vi "Estimated Time Required.vi"(1 "Lithography Information":T1(array[cluster])) -> (0 "Estimated Time Required":timestamp format="%<%I:%M:%S>T")   [LabVIEW 2011]
doc: "Calculates the time required to complete lithography."
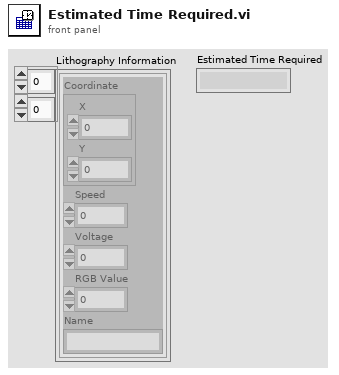
[diagram p1: front panel]
types:
  T1 = cluster{"Coordinate":cluster{"X":dbl, "Y":dbl}, "Speed":dbl, "Voltage":dbl, "RGB Value":i32, "Name":string}[][]
  T2 = cluster{"Coordinate":cluster{"X":dbl, "Y":dbl}, "Speed":dbl, "Voltage":dbl, "RGB Value":i32, "Name":string}
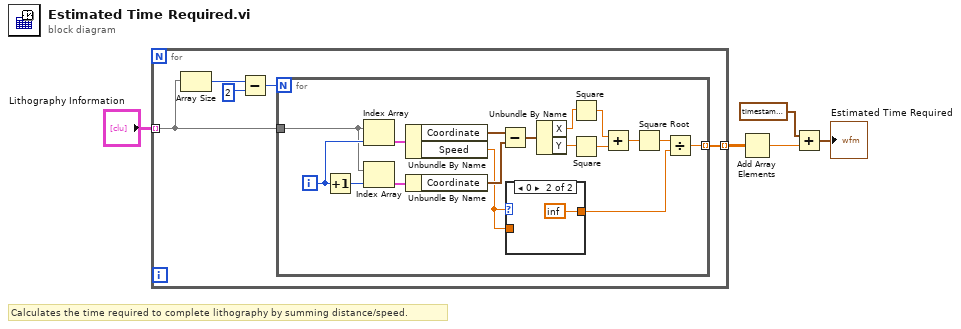
[diagram p0: block diagram]
diagram:
  # "Calculates the time required to complete lithography by summing distance/speed."
  n1 = for {
    tunnel: "Lithography Information" -> [w10] mode=indexing
    tunnel: [w9] -> w4 mode=indexing
    n2 = Array Size(array=w10) -> (size(s)=w7:i32)
    n3 = Subtract(x=w7, y=2) -> (x-y=w6:i32)
    n4 = for {
      N: w6 -> [_]
      tunnel: w10 -> [w25]
      tunnel: [w13] -> w9 mode=indexing
      i -> [w26]
      n5 = Increment(x=w26) -> (x+1=w27:i32)
      n6 = Index Array(array=w25, index=w26) -> (element=w23:T2)
      n7 = Index Array(array=w25, index=w27) -> (element=w24:T2)
      n8 = Unbundle By Name(w23) -> ("Coordinate"=w21:cluster{"X":dbl, "Y":dbl}, "Speed"=w12:dbl)
      n9 = Unbundle By Name(w24) -> ("Coordinate"=w22:cluster{"X":dbl, "Y":dbl})
      n10 = Subtract(x=w21, y=w22) -> (x-y=w20:cluster{"X":dbl, "Y":dbl})
      n11 = case shown="0" w12 {
        tunnel: w12 -> [w28 _]
        tunnel: [w28 inf] -> w11
        frame 1, Default {
        }
        frame 0 {
        }
      }
      n12 = Unbundle By Name(w20) -> ("X"=w19:dbl, "Y"=w18:dbl)
      n13 = Square(x=w19) -> (x^2=w17:dbl)
      n14 = Square(x=w18) -> (x^2=w16:dbl)
      n15 = Add(x=w17, y=w16) -> (x+y=w15:dbl)
      n16 = Square Root(x=w15) -> (sqrt(x)=w14:dbl)
      n17 = Divide(x=w14, y=w11) -> (x/y=w13:dbl)
    }
  }
  n18 = Add Array Elements(numeric array=w4) -> (sum=w2:dbl)
  n19 = Add(x=timestamp(-68400 s since 1904-01-01), y=w2) -> (x+y=→"Estimated Time Required":timestamp)
